vi "Create_Experiment_Information_File.vi"(3 "error in":errorcluster, 4 "Time Elapsed":string, 5 "Folder path in":path, 6 "Data in":T1={"User Name"="", "Experiment Number"=0, "Start Time"=timestamp(0 s since 1904-01-01), "Data"=[], "Step Number"=1, "Step Instructions"="", "Diagnostics"={"Langmuir Probe"=FALSE, "Rogowski 1"=FALSE, "Rogowski 2"=FALSE, "Rogowski 3"=FALSE, "B-dot 1"=FALSE, "B-dot 2"=FALSE}, "Experiment Purpose"="", "Experiment State"=enum."Off", "Systems"={"Compressed Air"=FALSE, "T-20kV Power Switch"=FALSE, "T-Rectifier"=FALSE, "Engage Interlock"=FALSE, "Ventilator"=FALSE, "Magnetron"=FALSE, "H-20kV Power Switch"=FALSE, "H-Rectifier"=FALSE, "Main Water Pump"=FALSE, "WEGA Water Pump"=FALSE, "Gas Inlet Valves"=FALSE}, "Current Pressure"=0.0, "Fieldpoints"={"System Boolean Fieldpoints"={"Compressed Air"="", "T-20kV Power Switch"="", "T-Rectifier"="", "Engage Interlock"="", "Ventilator"="", "Magnetron"="", "H-20kV Power Switch"="", "H-Rectifier"="", "Main Water Pump"="", "WEGA Water Pump"="", "Gas Inlet Valves"=""}, "Step Fieldpoints"={"Exhaust Ventillator"="", "Compressed Air"="", "Water Pressure"="", "Interlock"="", "Toroidal Power Supply 1"="", "Toroidal Power Supply 2"="", "Toroidal Rectifier"="", "Helical Power Supply"="", "Helical Rectifier"="", "6kW Magnetron Standby"="", "20kW Magnetron Standby"=""}}, "Pressure History"={"Seconds into Experiment"=[], "Pressure Data"=[]}}) -> (0 "error out":errorcluster, 1 "Folder path out":path, 2 "Data out":T1={"User Name"="", "Experiment Number"=0, "Start Time"=timestamp(0 s since 1904-01-01), "Data"=[], "Step Number"=1, "Step Instructions"="", "Diagnostics"={"Langmuir Probe"=FALSE, "Rogowski 1"=FALSE, "Rogowski 2"=FALSE, "Rogowski 3"=FALSE, "B-dot 1"=FALSE, "B-dot 2"=FALSE}, "Experiment Purpose"="", "Experiment State"=enum."Off", "Systems"={"Compressed Air"=FALSE, "T-20kV Power Switch"=FALSE, "T-Rectifier"=FALSE, "Engage Interlock"=FALSE, "Ventilator"=FALSE, "Magnetron"=FALSE, "H-20kV Power Switch"=FALSE, "H-Rectifier"=FALSE, "Main Water Pump"=FALSE, "WEGA Water Pump"=FALSE, "Gas Inlet Valves"=FALSE}, "Current Pressure"=0.0, "Fieldpoints"={"System Boolean Fieldpoints"={"Compressed Air"="", "T-20kV Power Switch"="", "T-Rectifier"="", "Engage Interlock"="", "Ventilator"="", "Magnetron"="", "H-20kV Power Switch"="", "H-Rectifier"="", "Main Water Pump"="", "WEGA Water Pump"="", "Gas Inlet Valves"=""}, "Step Fieldpoints"={"Exhaust Ventillator"="", "Compressed Air"="", "Water Pressure"="", "Interlock"="", "Toroidal Power Supply 1"="", "Toroidal Power Supply 2"="", "Toroidal Rectifier"="", "Helical Power Supply"="", "Helical Rectifier"="", "6kW Magnetron Standby"="", "20kW Magnetron Standby"=""}}, "Pressure History"={"Seconds into Experiment"=[], "Pressure Data"=[]}})   [LabVIEW 2015]
uses:
  Type_Defs/Data.ctl
  Type_Defs/Diagnostics.ctl
  Type_Defs/Systems.ctl
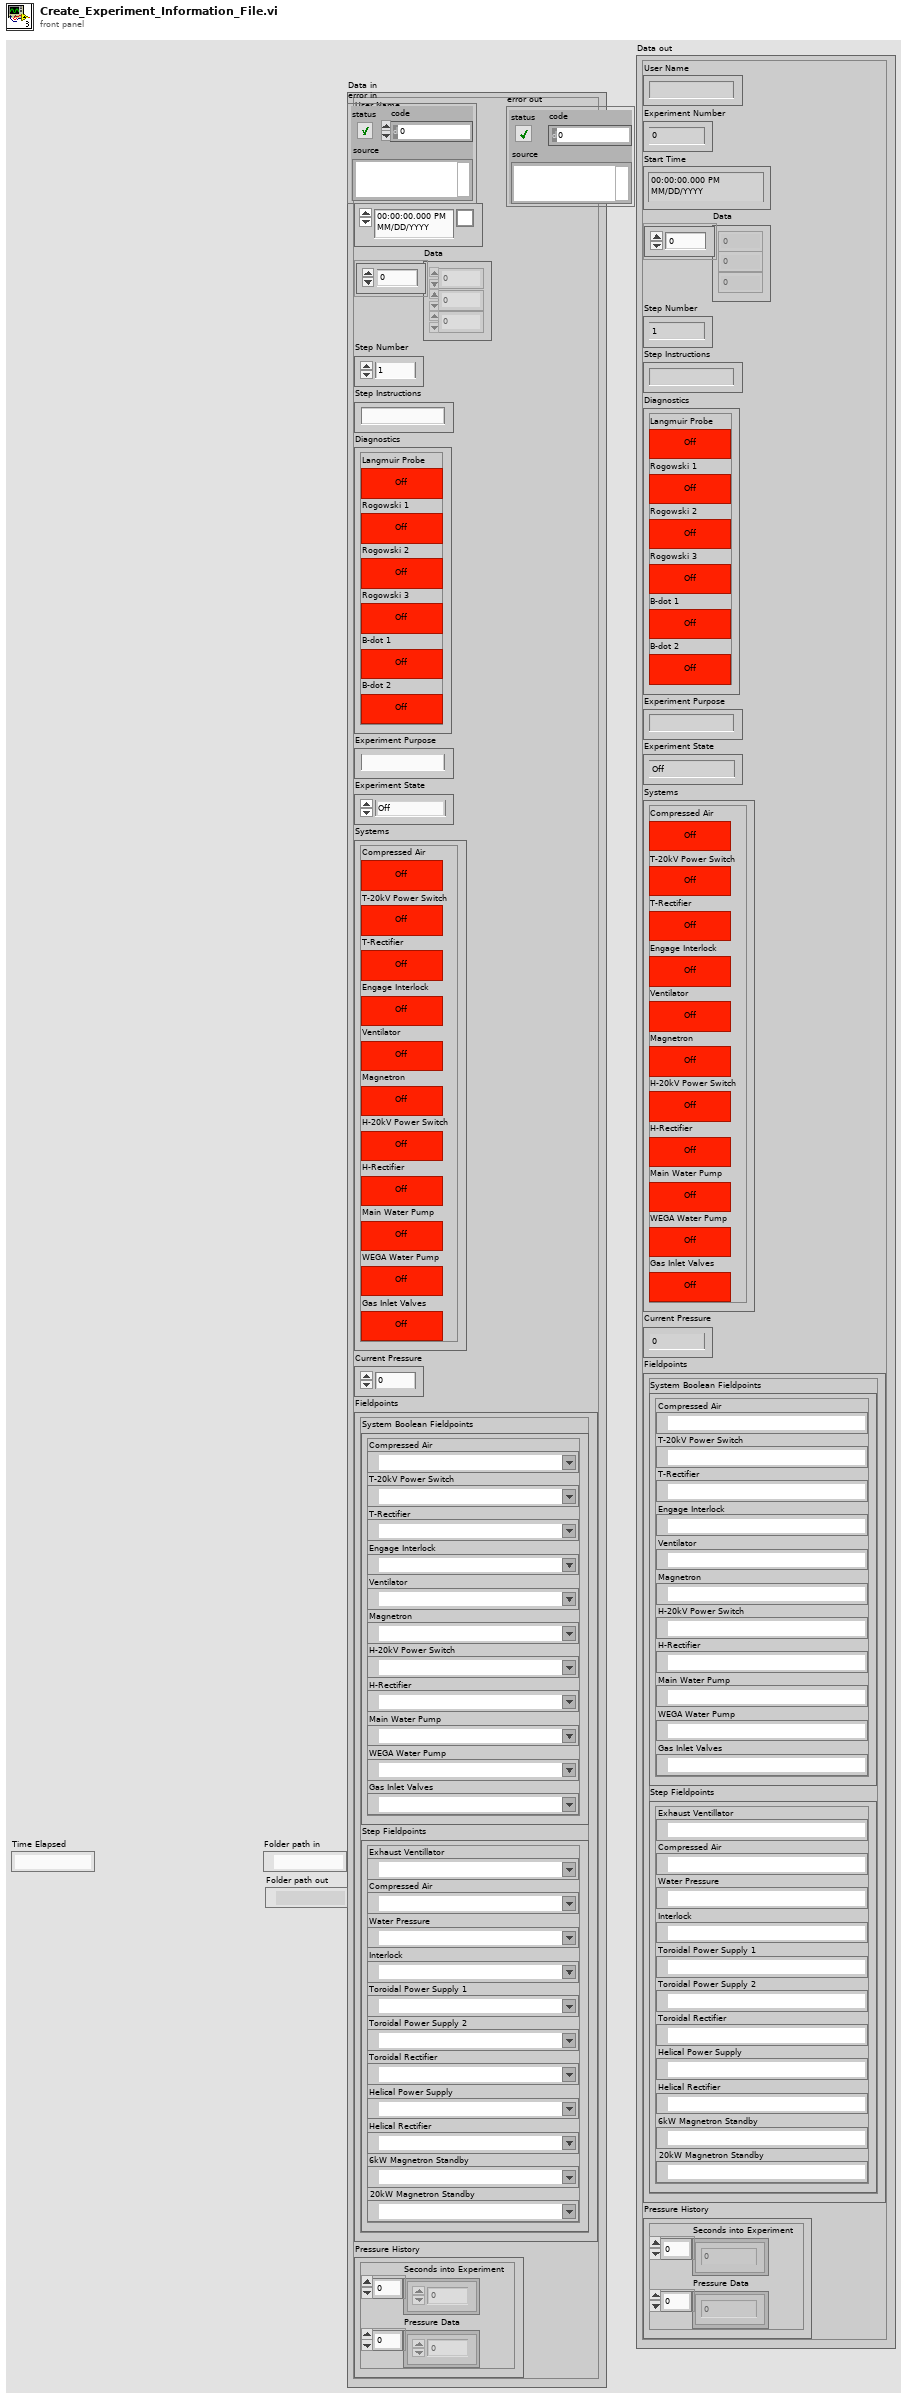
[diagram p1: front panel]
types:
  T1 = typedef "Data.ctl" = cluster{"User Name":string, "Experiment Number":i32, "Start Time":timestamp, "Data":dbl[], "Step Number":i32, "Step Instructions":string, "Diagnostics":T2, "Experiment Purpose":string, "Experiment State":enum16{"Off", "Setting Up", "Ready", "In Progress", "Shutting Down"}, "Systems":T3, "Current Pressure":dbl, "Fieldpoints":cluster{"System Boolean Fieldpoints":cluster{"Compressed Air":refnum<k21>, "T-20kV Power Switch":refnum<k21>, "T-Rectifier":refnum<k21>, "Engage Interlock":refnum<k21>, "Ventilator":refnum<k21>, "Magnetron":refnum<k21>, "H-20kV Power Switch":refnum<k21>, "H-Rectifier":refnum<k21>, "Main Water Pump":refnum<k21>, "WEGA Water Pump":refnum<k21>, "Gas Inlet Valves":refnum<k21>}, "Step Fieldpoints":cluster{"Exhaust Ventillator":refnum<k21>, "Compressed Air":refnum<k21>, "Water Pressure":refnum<k21>, "Interlock":refnum<k21>, "Toroidal Power Supply 1":refnum<k21>, "Toroidal Power Supply 2":refnum<k21>, "Toroidal Rectifier":refnum<k21>, "Helical Power Supply":refnum<k21>, "Helical Rectifier":refnum<k21>, "6kW Magnetron Standby":refnum<k21>, "20kW Magnetron Standby":refnum<k21>}}, "Pressure History":cluster{"Seconds into Experiment":i32[], "Pressure Data":dbl[]}}
  T2 = typedef "Diagnostics.ctl" = cluster{"Langmuir Probe":bool, "Rogowski 1":bool, "Rogowski 2":bool, "Rogowski 3":bool, "B-dot 1":bool, "B-dot 2":bool}
  T3 = typedef "Systems.ctl" = cluster{"Compressed Air":bool, "T-20kV Power Switch":bool, "T-Rectifier":bool, "Engage Interlock":bool, "Ventilator":bool, "Magnetron":bool, "H-20kV Power Switch":bool, "H-Rectifier":bool, "Main Water Pump":bool, "WEGA Water Pump":bool, "Gas Inlet Valves":bool}
  T4 = enum16{"open", "replace", "create", "open or create", "replace or create", "replace or create with confirmation"}
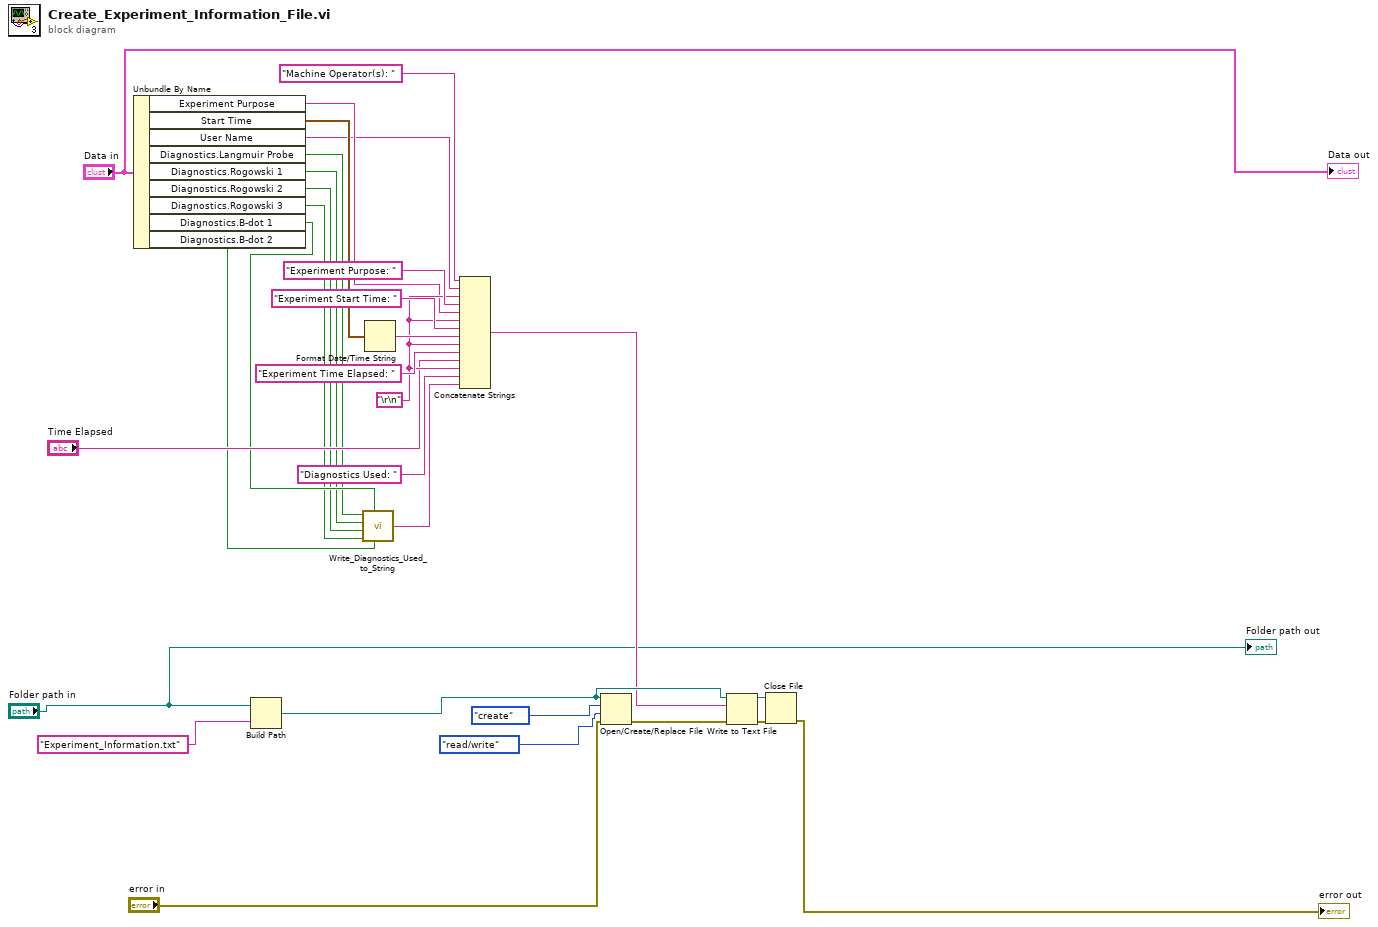
[diagram p0: block diagram]
diagram:
  w16 = "\r\n"
  n1 = Unbundle By Name("Data in") -> ("Experiment Purpose"=w15:string, "Start Time"=w14:timestamp, "User Name"=w5:string, "Diagnostics.Langmuir Probe"=w10:bool, "Diagnostics.Rogowski 1"=w9:bool, "Diagnostics.Rogowski 2"=w8:bool, "Diagnostics.Rogowski 3"=w7:bool, "Diagnostics.B-dot 1"=w11:bool, "Diagnostics.B-dot 2"=w6:bool)
  n2 = Build Path(base path="Folder path in", name or relative path="Experiment_Information.txt" ("string")) -> (appended path=w24:path)
  n3 = call "Write_Diagnostics_Used_to_String.vi"("| B-dot 2 |"=w6, "| B-dot 1 |"=w11, "| Rogowski 3 |"=w7, "| Rogowski 2 |"=w8, "| Rogowski 1 |"=w9, "| Lanmuir Probe |"=w10) -> ("String"=w12:string)
  n4 = Format Date/Time String(seconds (now)=w14) -> (date/time string=w21:string)  [unwired: 2 in]
  n5 = Concatenate Strings("Machine Operator(s): " ("string"), w5, w16, "Experiment Purpose: " ("string"), w15, w16, "Experiment Start Time: " ("string"), w21, w16, "Experiment Time Elapsed: " ("string"), "Time Elapsed", w16, "Diagnostics Used: " ("string"), w12) -> (w4:string)
  n6 = Open/Create/Replace File(file path (use dialog)=w24, error in="error in", operation (0:open)=T4."create", access (0:read/write)=enum16{"read/write", "read-only", "write-only"}."read/write") -> (error out=w27:errorcluster)  [unwired: 2 in, 2 out]
  n7 = Write to Text File(file (use dialog)=w24, text=w4, error in=w27) -> (refnum out=w29:refnum<file>, error out=w28:errorcluster)  [unwired: 1 in, 1 out]
  n8 = Close File(refnum=w29, error in=w28) -> (error out=→"error out":errorcluster)  [unwired: 1 out]
  "Data out" <- "Data in"
  "Folder path out" <- "Folder path in"
